vi "Close App.vi"(8 "error in (no error)":errorcluster, 11 "Application in":refnum<class "Application.lvclass">) -> (0 "error out":errorcluster)   [LabVIEW 2021, in "Application.lvclass"]
uses:
  Application.lvclass
  <vilib>/event_ctls.llb/usereventprio.ctl
  Application.lvclass/Application.ctl
  Board Game_class/Board Game.lvclass/Board Game.ctl
  Board Game_class/Read Bomb.vi
  Board Game_class/Read Shield.vi
  Board Game_class/Read Snake.vi
  Board Game_class/Read Fruit.vi
  Bomb/Bomb.lvclass
  C:/Users/poche/Programs/LabVIEW/imposible snake/GameEl_class/GameEl.lvclass
  Shield/Shield.lvclass
  Snake_class/Snake.lvclass
  Fruit_class/Fruit.lvclass
  GameEl_class/GameEl.lvclass
  Board Game_class/Board Game.lvclass
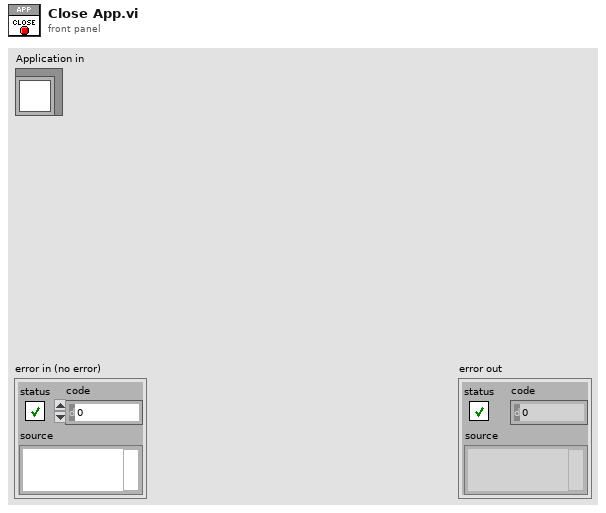
[diagram p1: front panel]
types:
  T1 = typedef "usereventprio.ctl" = enum32{"high priority", "normal priority"}
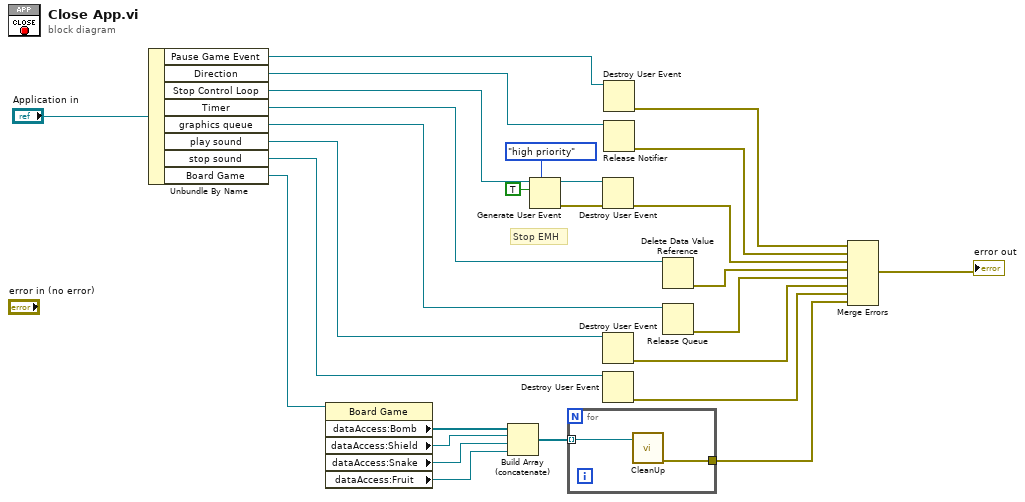
[diagram p0: block diagram]
diagram:
  # "Stop EMH"
  n1 = Unbundle By Name("Application in") -> ("Pause Game Event"=w22:refnum<user-event>, "Direction"=w23:refnum<notifier>, "Stop Control Loop"=w24:refnum<user-event>, "Timer"=w17:refnum<data-value>, "graphics queue"=w13:refnum<queue>, "play sound"=w4:refnum<user-event>, "stop sound"=w3:refnum<user-event>, "Board Game"=w10:refnum<class "Board Game.lvclass">)
  n2 = property class="Board Game"(reference=w10) -> ("dataAccess:Bomb"=w9:refnum<class "Bomb.lvclass">[], "dataAccess:Shield"=w8:refnum<class "Shield.lvclass">, "dataAccess:Snake"=w7:refnum<class "Snake.lvclass">, "dataAccess:Fruit"=w6:refnum<class "Fruit.lvclass">)  [unwired: 1 in, 2 out]
  n3 = Build Array (concatenate)(w9, w8, w7, w6) -> (w5:refnum<class "GameEl.lvclass">[])
  n4 = Generate User Event(priority (normal)=usereventprio."high priority", user event=w24, event data cluster=TRUE ("event data")) -> (user event out=w25:refnum<user-event>, error out=w21:errorcluster)  [unwired: 1 in]
  n5 = for {
    tunnel: w5 -> [w29] mode=indexing
    tunnel: [w28] -> w2
    n6 = call-dynamic "CleanUp.vi"("object in"=w29) -> ("Error Out"=w28:errorcluster)  [unwired: 9 in, 1 out]
  }
  n7 = Destroy User Event(user event=w25, error in=w21) -> (error out=w18:errorcluster)
  n8 = Destroy User Event(user event=w4) -> (error out=w11:errorcluster)  [unwired: 1 in]
  n9 = Destroy User Event(user event=w3) -> (error out=w1:errorcluster)  [unwired: 1 in]
  n10 = Destroy User Event(user event=w22) -> (error out=w20:errorcluster)  [unwired: 1 in]
  n11 = Release Notifier(notifier=w23) -> (error out=w19:errorcluster)  [unwired: 2 in, 2 out]
  n12 = Delete Data Value Reference(data value reference=w17) -> (error out=w16:errorcluster)  [unwired: 1 in, 1 out]
  n13 = Release Queue(queue=w13) -> (error out=w12:errorcluster)  [unwired: 2 in, 2 out]
  n14 = Merge Errors(w20, w19, w18, w16, w12, w11, w1, w2) -> (→"error out":errorcluster)
